vi "Upper Target Loop.vi"(11 "Camera Name":string="cam0") -> ()   [LabVIEW 2020]
uses:
  Camera Types.ctl
  Utilities/Camera Setup Cluster.ctl
  <vilib>/vision/Image Controls.llb/IMAQ Image.ctl
  Camera Set Up/Event Setup Types.ctl
  <vilib>/Utility/config.llb/Write Key (String).vi
  <vilib>/Utility/config.llb/Read Key (String).vi
  <vilib>/vision/NI_Vision_Development_Module.lvlib
  <vilib>/Utility/config.llb/NI_LVConfig.lvlib
panel:
  in  "Main":enum32{"Page 1", "Page 2"}(tab)
  in  "Configure":bool
  in  "Brightness":i32=50 min=0 max=100
  in  "Camera":enum32{"Mask", "Image With Target"}(tab)
  out "Mask":T1(plugin-control)
  out "Image":T1(plugin-control)
  in  "Save":bool
  out "Angle Array":dbl[](array[numeric]) format="%.1f"
  out "Distance  Array":dbl[](array[numeric]) format="%.1f"
  in  "White Balance":T2(ring)=enum."Fixed indoor"
  in  "FOV":dbl=120.0
  in  "Size Limit %":dbl=0.02 format="%#_13g"
  in  "Home":bool
  in  "Color Range":T3={"Hue"={21.620689392089844, 69.62068939208984}, "Sat"={66.41378784179688, 255.0}, "Val"={96.0, 255.0}} {"Hue" scale=0.0..255.0 scale format="%#_3g"}
  out "Fps":dbl format="%#.0f"
  in  "Camera Type":T4=enum."MS HD3000 640x480"
  in  "Dilate":bool
  in  "Robot Calibration":T5={"Camera Height on robot (in)"=26.7, "Camera Angle on the robot (deg)"=21.6, "Slope"=0.946, "Offset"=10.775} {"Offset" format="%#_13g"; "Slope" format="%#_13g"; "Camera Angle on the robot (deg)" format="%#_13g"; "Camera Height on robot (in)" format="%#_13g"}
  in  "Camera Exposure":i64=50 min=1 max=100
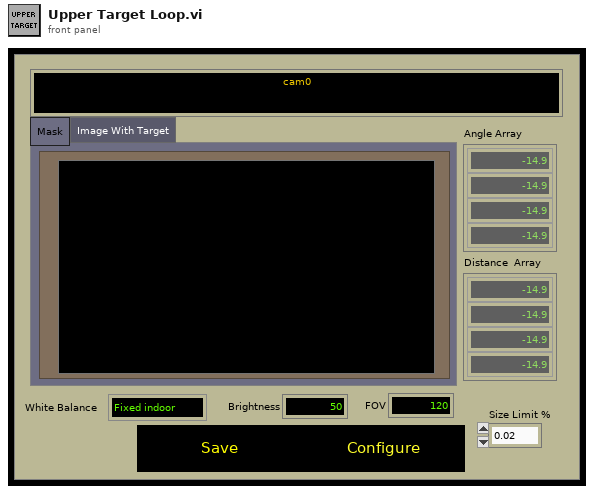
[diagram p1: front panel]
types:
  T1 = typedef "IMAQ Image.ctl" = refnum<image>
  T2 = enum16{"Auto", "Fixed indoor", "Fixed outdoor 1", "Fixed outdoor 2", "Fixed fluorescent 1", "Fixed fluorescent 2", "Hold current", "Custom"}
  T3 = cluster{"Hue":cluster{dbl, dbl}, "Sat":cluster{dbl, dbl}, "Val":cluster{dbl, dbl}}
  T4 = typedef "Camera Types.ctl" = enum16{"206", "1011", "1013", "MS HD3000 square", "MS HD3000 640x480", "MS HD3000 1280x720"}
  T5 = typedef "Camera Setup Cluster.ctl" = cluster{"Camera Height on robot (in)":dbl, "Camera Angle on the robot (deg)":dbl, "Slope":dbl, "Offset":dbl}
  T6 = typedef "Image Type" = u32
  T7 = typedef "Particle Parameters" = i32
  T8 = enum32{"AutoM", "Close", "Dilate", "Erode", "Gradient", "Gradient out", "Gradient in", "Hit miss", "Open", "PClose", "POpen", "Thick", "Thin"}
  T9 = typedef "Event Setup Types.ctl" = enum16{"Save Data", "Calibrate", "Set White Balance", "Set Brightness", "Set Exposure", "Update Brightness", "Update Exposure", "Update White Balance", "Exit"}
  T10 = typedef "Target Fields.ctl" = cluster{"diameter points":cluster{"first point":cluster{"x":dbl, "y":dbl}, "projected point":cluster{"x":dbl, "y":dbl}}, "normalized center":cluster{"x":dbl, "y":dbl}, "Overall Score":dbl, "Area Score":dbl, "Moment Score":dbl, "Aspect Score":dbl, "Distance (ft)":dbl, "Upper Goal":bool}
  T11 = typedef "NI_LVConfig.lvlib/Config Data RefNum.ctl" = refnum<k1>
  T12 = cluster{cluster{"Lower":dbl, "Upper":dbl}, cluster{"Lower":dbl, "Upper":dbl}, cluster{"Lower":dbl, "Upper":dbl}}
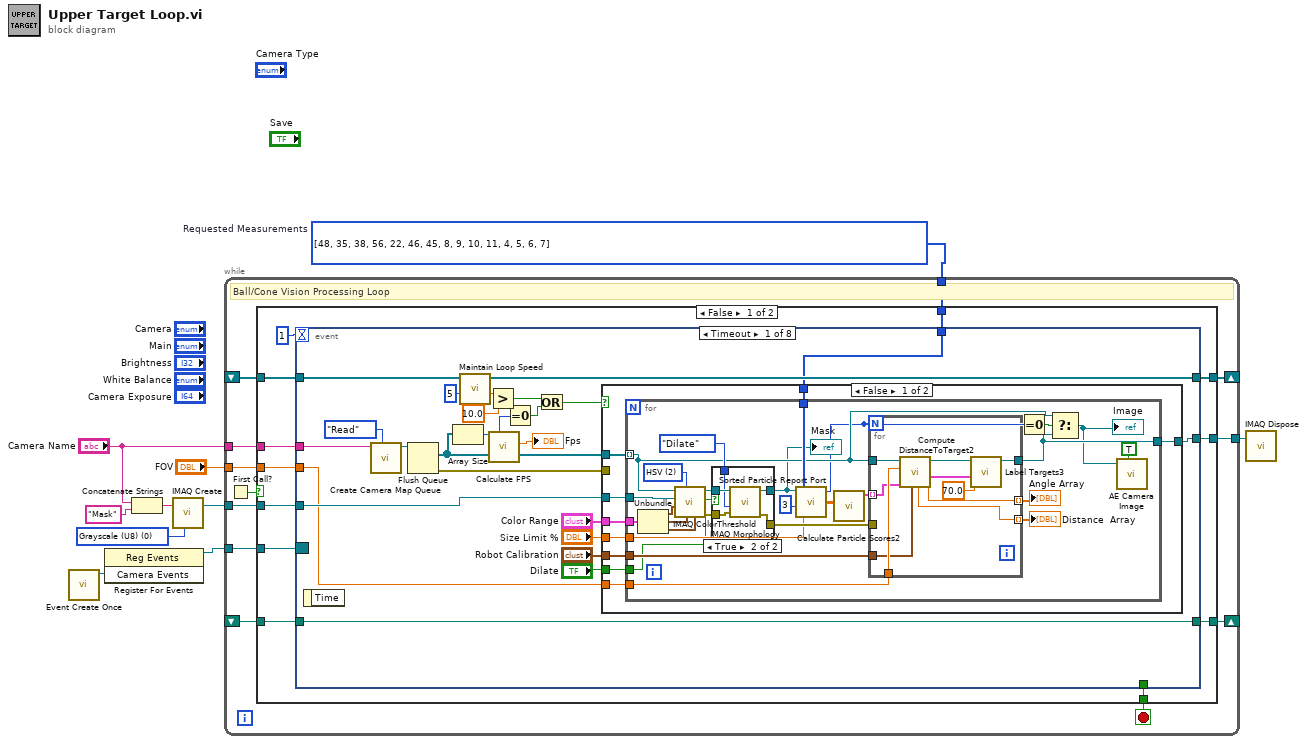
[diagram p0: block diagram]
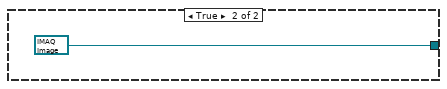
[diagram p3: hidden frame]
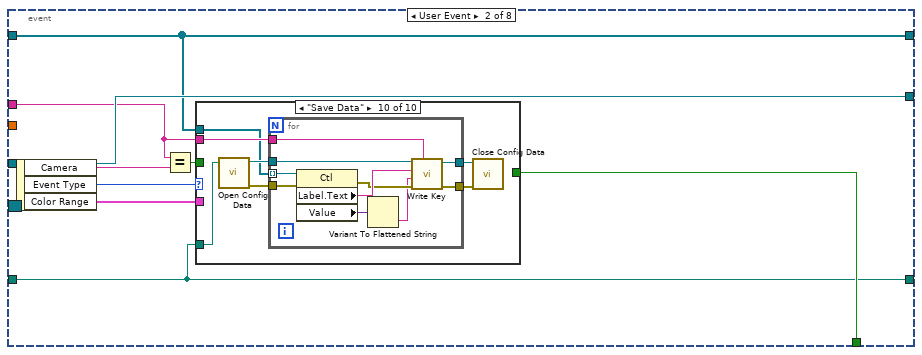
[diagram p4: hidden frame]
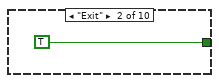
[diagram p6: hidden frame]
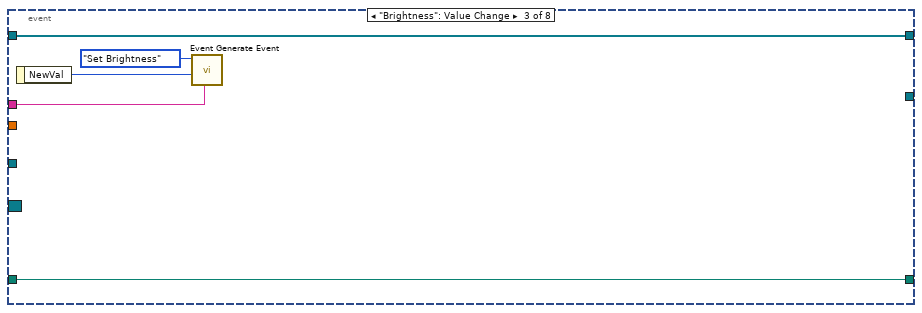
[diagram p14: hidden frame]
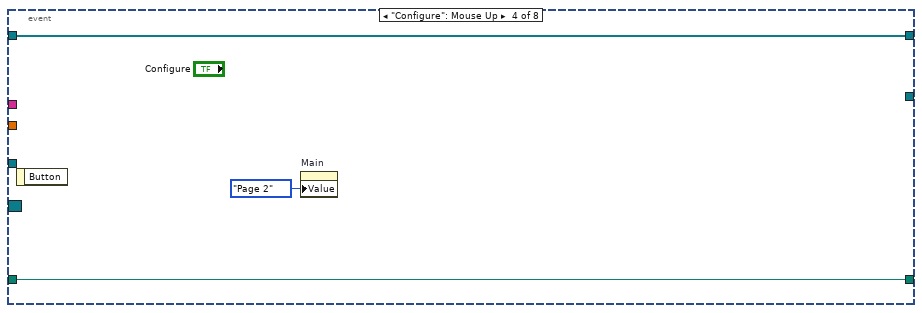
[diagram p15: hidden frame]
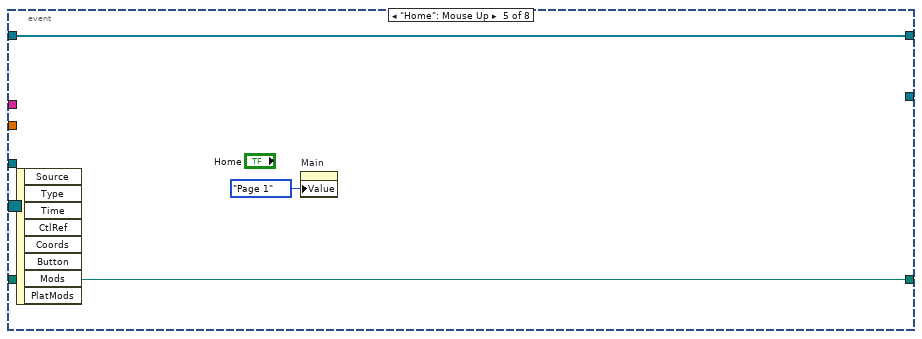
[diagram p16: hidden frame]
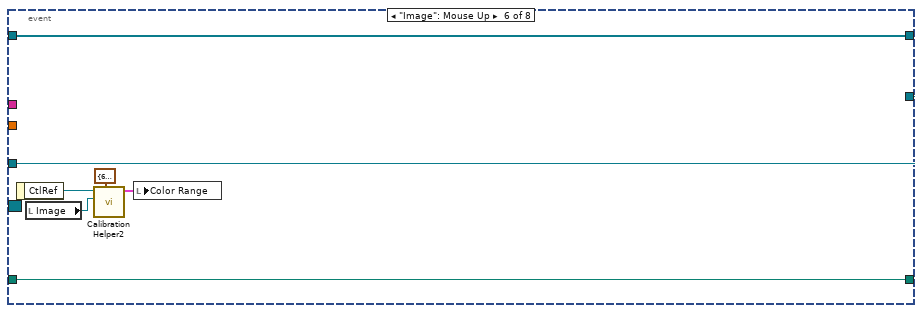
[diagram p17: hidden frame]
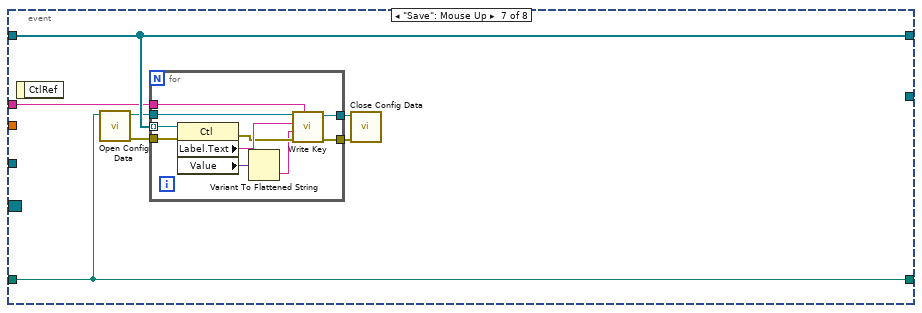
[diagram p18: hidden frame]
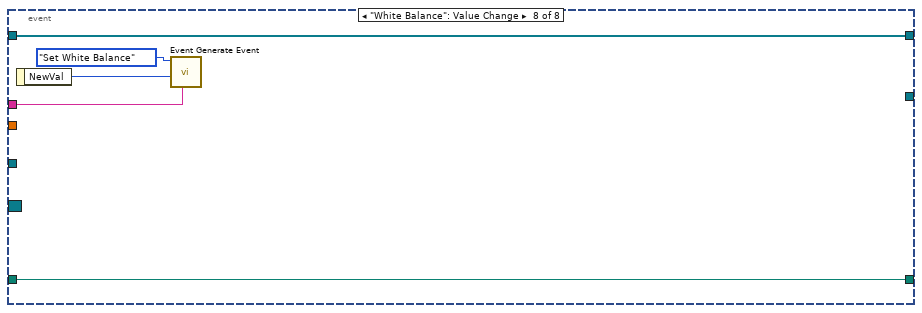
[diagram p19: hidden frame]
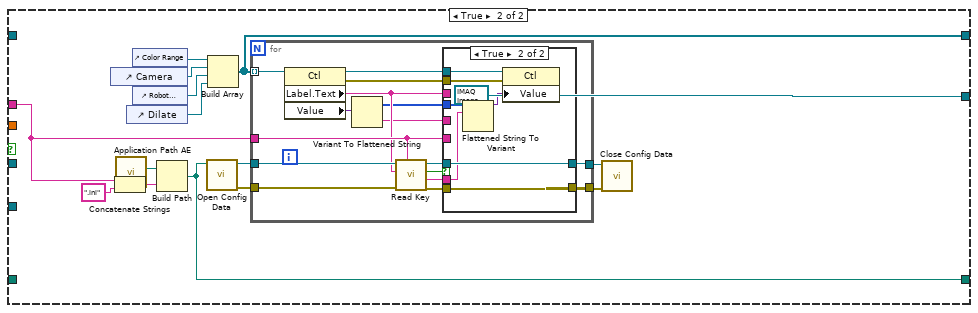
[diagram p20: hidden frame]
diagram:
  w6 = T6 0 items=["Grayscale (U8)", "Grayscale (I16)", "Grayscale (SGL)", "Complex (CSG)", "RGB (U32)", "HSL (U32)", "RGB (U64)", "Grayscale (U16)"] ("Image Type")
  w2 = T7[] [48, 35, 38, 56, 22, 46, 45, 8, 9, 10, 11, 4, 5, 6, 7] items=["Center of Mass X", "Center of Mass Y", "First Pixel X", "First Pixel Y", "Bounding Rect Left", "Bounding Rect Top", "Bounding Rect Right", "Bounding Rect Bottom", "Max Feret Diameter Start X", "Max Feret Diameter Start Y", "Max Feret Diameter End X", "Max Feret Diameter End Y", "Max Horiz. Segment Length Left", "Max Horiz. Segment Length Right", "Max Horiz. Segment Length Row", "-", "Bounding Rect Width", "Bounding Rect Height", "Bounding Rect Diagonal", "Perimeter", "Convex Hull Perimeter", "Holes' Perimeter", "Max Feret Diameter", "Equivalent Ellipse Major Axis", "Equivalent Ellipse Minor Axis", "Equivalent Ellipse Minor Axis (Feret)", "Equivalent Rect Long Side", "Equivalent Rect Short Side", "Equivalent Rect Diagonal", "Equivalent Rect Short Side (Feret)", "Average Horiz. Segment Length", "Average Vert. Segment Length", "Hydraulic Radius", "Waddel Disk Diameter", "-", "Area", "Holes' Area", "Particle & Holes' Area", "Convex Hull Area", "Image Area", "-", "Number of Holes", "Number of Horiz. Segments", "Number of Vert. Segments", "-", "Orientation", "Max Feret Diameter Orientation", "-", "% Area/Image Area", "% Area/(Particle & Holes' Area)", "Ratio of Equivalent Ellipse Axes", "Ratio of Equivalent Rect Sides", "-", "Elongation Factor", "Compactness Factor", "Heywood Circularity Factor", "Type Factor", "-", "Sum X", "Sum Y", "Sum XX", "Sum XY", "Sum YY", "Sum XXX", "Sum XXY", "Sum XYY", "Sum YYY", "-", "Moment of Inertia XX", "Moment of Inertia XY", "Moment of Inertia YY", "Moment of Inertia XXX", "Moment of Inertia XXY", "Moment of Inertia XYY", "Moment of Inertia YYY", "Norm. Moment of Inertia XX", "Norm. Moment of Inertia XY", "Norm. Moment of Inertia YY", "Norm. Moment of Inertia XXX", "Norm. Moment of Inertia XXY", "Norm. Moment of Inertia XYY", "Norm. Moment of Inertia YYY", "Hu Moment 1", "Hu Moment 2", "Hu Moment 3", "Hu Moment 4", "Hu Moment 5", "Hu Moment 6", "Hu Moment 7"]  # Requested Measurements
  n1 = call "Event Create Once.vi"() -> ("Camera Events"=w8:refnum<user-event>)  [unwired: 10 in, 1 out]
  n2 = register-events(w8) -> (reference out=w7:refnum<event-registration>)  [unwired: 2 in, 1 out]
  n3 = Concatenate Strings("Camera Name", "Mask" ("string")) -> (w5:string)
  n4 = call "IMAQ Create"("Image Name"=w5, "Image Type"=w6) -> ("New Image"=w10:T1)  [unwired: 2 in, 2 out]
  n5 = while {
    tunnel: w10 -> [w22]
    tunnel: w2 -> [w21]
    tunnel: [w20] -> w9
    tunnel: w7 -> [w19]
    tunnel: "FOV" -> [w17]
    tunnel: "Camera Name" -> [w16]
    shift-right: [w14] -> _
    shift-left: _ -> [w13]
    shift-right: [w12] -> _
    shift-left: _ -> [w11]
    stop <- w18 stop-if-true
    # "Ball/Cone Vision Processing Loop"
    n6 = First Call?() -> (First Call?: T/F=w15:bool)
    n7 = case shown="False" w15 {
      tunnel: w22 -> [w34 _]
      tunnel: w21 -> [w33 _]
      tunnel: [w32 T1 refnum ("New Image")] -> w20
      tunnel: w19 -> [w30 _]
      tunnel: [w29 _] -> w18
      tunnel: w17 -> [w28 _]
      tunnel: w16 -> [w27 w187]
      tunnel: [w25 w186] -> w14
      tunnel: w13 -> [w26 _]
      tunnel: [w23 w185] -> w12
      tunnel: w11 -> [w24 _]
      frame False {
        n8 = event shown="[0] Timeout" {
          selector: w30 -> [_ _ _ _ _ _ _ _]
          dyn-events: _ -> [_ _ _ _ _ _ _ _]
          timeout: 1 -> [_ _ _ _ _ _ _ _]
          tunnel: w34 -> [w51 w120 _ _ _ w154 _ _]
          tunnel: w33 -> [w49 _ _ _ _ _ _ _]
          tunnel: [w47 w120 _ _ _ w154 _ _] -> w32
          tunnel: [_ w118 _ _ _ _ _ _] -> w29
          tunnel: w28 -> [w50 _ _ _ _ _ _ _]
          tunnel: w27 -> [w56 w114 w141 _ _ _ w161 w176]
          tunnel: w26 -> [w55 w112 w140 w146 w149 w153 w162 w175]
          tunnel: [w55 w112 w140 w146 w149 w153 w162 w175] -> w25
          tunnel: w24 -> [w54 w113 w139 w145 w148 w152 w163 w174]
          tunnel: [w54 w113 w139 w145 w148 w152 w163 w174] -> w23
          event Timeout {
            n9 = event-data() -> ()  [unwired: 1 in, 1 out]
            n10 = call "Create Camera Map Queue.vi"("Action"=enum16{"Read", "Write"}."Read", "key"=w56) -> ("value"=w41:refnum<queue>)  [unwired: 8 in, 1 out]
            n11 = Flush Queue(queue=w41) -> (remaining elements=w36:T1[], error out=w40:errorcluster)  [unwired: 1 in, 1 out]
            n12 = Array Size(array=w36) -> (size(s)=w39:i32)
            n13 = call "Maintain Loop Speed.vi"("setpoint (msec)"=5) -> ("Loop Time"=w44:dbl)  [unwired: 10 in]
            n14 = Greater?(x=w44, y=10.0) -> (0:w45:bool)
            n15 = call "Calculate FPS.vi"("Frames Processed"=w39) -> ("Fps"=→"Fps":dbl)  [unwired: 10 in]
            n16 = Equal To 0?(x=w39) -> (x = 0?=w46:bool)
            n17 = Or(x=w45, y=w46) -> (x .or. y?=w35:bool)
            n18 = case shown="False" w35 {
              tunnel: w49 -> [w66 _]
              tunnel: w51 -> [w65 _]
              tunnel: [w60 T1 refnum ("Image out")] -> w47
              tunnel: "Color Range" -> [w64 _]
              tunnel: "Size Limit %" -> [w63 _]
              tunnel: "Robot Calibration" -> [w62 _]
              tunnel: w50 -> [w61 _]
              tunnel: "Dilate" -> [w59 _]
              tunnel: w36 -> [w58 _]
              tunnel: w40 -> [_ _]
              frame False {
                n19 = for {
                  tunnel: w66 -> [w93]
                  tunnel: w65 -> [w89]
                  tunnel: [w85] -> w60
                  tunnel: w58 -> [w78] mode=indexing
                  tunnel: w64 -> [w77]
                  tunnel: w63 -> [w76]
                  tunnel: w62 -> [w75]
                  tunnel: w61 -> [w74]
                  tunnel: w59 -> [w71]
                  w83 = u16 2 items=["RGB", "HSL", "HSV", "HSI"] ("Color Mode")
                  n20 = Unbundle(w77) -> ("Hue"=w90:cluster{dbl, dbl}, "Sat"=w92:cluster{dbl, dbl}, "Val"=w91:cluster{dbl, dbl})
                  n21 = call "IMAQ ColorThreshold"("Blue or Luma or Val or Inten Range"=w91, "Green or Sat Range"=w92, "Color Mode"=w83, "Red or Hue Range"=w90, "Image Dst"=w89, "Image Src"=w78) -> ("error out"=w80:errorcluster, "Image Dst Out"=w82:T1)  [unwired: 4 in]
                  n22 = case shown="True" w71 {
                    tunnel: w82 -> [w95 w100]
                    tunnel: [w95 w99] -> w70
                    tunnel: T8."Dilate" ("Operation") -> [_ w98]
                    tunnel: w80 -> [w94 w97]
                    tunnel: [w94 w96] -> w79
                    frame False {
                    }
                    frame True {
                      n23 = call "IMAQ Morphology"("error in (no error)"=w97, "Operation"=w98, "Image Src"=w100) -> ("error out"=w96:errorcluster, "Image Dst Out"=w99:T1)  [unwired: 7 in]
                    }
                  }
                  "Mask" <- w70
                  n24 = call "Sorted Particle Report Port.vi"("Min Area Size %"=w76, "Particle Count Limit"=3 ("Particle Count"), "Pixel Measurements"=w93, "Image in"=w70) -> ("Sorted Data"=w87:dbl[][], "Particles"=w73:i32)  [unwired: 1 out]
                  n25 = call "Calculate Particle Scores2.vi"("Sorted Data"=w87) -> ("Scores"=w86:T10[])  [unwired: 10 in]
                  n26 = for {
                    N: w73 -> [_]
                    tunnel: w86 -> [w105] mode=indexing
                    tunnel: [w104] -> w68 mode=indexing
                    tunnel: w74 -> [w106]
                    tunnel: w75 -> [w103]
                    tunnel: w79 -> [_]
                    tunnel: w78 -> [w109]
                    tunnel: [w110] -> w85
                    tunnel: [w101] -> w67 mode=indexing
                    n27 = call "Compute DistanceToTarget2.vi"("Robot Calibration Cluster"=w103, "results"=w105, "Field of view"=w106, "Image Src"=w109) -> ("results out"=w107:T10, "Offset Angle"=w104:dbl, "Image Dst Out"=w108:T1, "DIstance"=w101:dbl)  [unwired: 3 in, 1 out]
                    n28 = call "Label Targets3.vi"("Score Threshold"=70.0 ("Score Threshold %"), "results"=w107, "Image in"=w108) -> ("Image out"=w110:T1)  [unwired: 8 in]
                  }
                  "Angle Array" <- w68
                  "Distance  Array" <- w67
                  n29 = Equal To 0?(x=w73) -> (x = 0?=w84:bool)
                  n30 = Select(t=w78, s=w84, f=w85) -> (s? t:f=w69:T1)
                  "Image" <- w69
                  n31 = call "AE Camera Image.vi"("Update"=TRUE, "Upper Image in"=w69) -> ()  [unwired: 9 in, 1 out]
                }
              }
              frame True {
              }
            }
          }
          event User Event {
            n32 = event-data() -> ("Camera"=w115:string, "Event Type"=w119:T9, "Color Range"=w116:T3)  [unwired: 1 in]
            n33 = Equal?(x=w114, y=w115) -> (x = y?=w117:bool)
            n34 = case shown="\"Save Data\"" w119 {
              tunnel: [_ TRUE _ _ _ _ _ _ _ _] -> w118
              tunnel: w117 -> [_ _ _ _ _ _ _ _ _ _]
              tunnel: w116 -> [_ _ _ _ _ _ _ _ _ _]
              tunnel: w114 -> [_ _ _ _ _ _ _ _ _ w124]
              tunnel: w113 -> [_ _ _ _ _ _ _ _ _ w123]
              tunnel: w112 -> [_ _ _ _ _ _ _ _ _ w122]
              frame Default {
              }
              frame "Exit" {
              }
              frame "Update White Balance" {
              }
              frame "Update Exposure" {
              }
              frame "Update Brightness" {
              }
              frame "Set Exposure" {
              }
              frame "Set Brightness" {
              }
              frame "Set White Balance" {
              }
              frame "Calibrate" {
              }
              frame "Save Data" {
                n35 = call <vilib>:"Open Config Data.vi"("configuration file path"=w123) -> ("error out"=w125:errorcluster, "refnum"=w128:T11)  [unwired: 8 in, 1 out]
                n36 = for {
                  tunnel: w122 -> [w136] mode=indexing
                  tunnel: w128 -> [w138]
                  tunnel: w124 -> [w137]
                  tunnel: [w133] -> w127
                  tunnel: [w131] -> w126
                  tunnel: w125 -> [w130]
                  n37 = property class="Ctl"(reference=w136, error in=w130) -> (error out=w132:errorcluster, "Label.Text"=w135:string, "Value"=w134:variant)  [unwired: 1 out]
                  n38 = Variant To Flattened String(Variant=w134) -> (data string=w129:string)  [unwired: 1 out]
                  n39 = call-poly <vilib>:"Write Key.vi"("section"=w137, "error in (no error)"=w132, "value"=w129, "key"=w135, "refnum"=w138) -> ("error out"=w131:errorcluster, "refnum out"=w133:T11)  [unwired: 4 in, 1 out]
                }
                n40 = call <vilib>:"Close Config Data.vi"("error in (no error)"=w126, "refnum"=w127) -> ()  [unwired: 8 in, 2 out]
              }
            }
          }
          event "Brightness": Value Change {
            n41 = event-data() -> ("NewVal"=w142:i32)  [unwired: 1 in]
            n42 = call "Event Generate Event.vi"("Camera"=w141, "Setpoint"=w142, "Event Type"=Event_Setup_Types."Set Brightness") -> ()  [unwired: 9 in]
          }
          event "Configure": Mouse Up {
            n43 = event-data() -> ()  [unwired: 1 in, 1 out]
            n44 = property on="Main" class="TabCtl (strict)"("Value"=enum32{"Page 1", "Page 2"}."Page 2" ("Main")) -> ()  [unwired: 2 in, 2 out]
          }
          event "Home": Mouse Up {
            n45 = event-data() -> ()  [unwired: 1 in, 8 out]
            n46 = property on="Main" class="TabCtl (strict)"("Value"=enum32{"Page 1", "Page 2"}."Page 1" ("Main")) -> ()  [unwired: 2 in, 2 out]
          }
          event "Image": Mouse Up {
            n47 = event-data() -> ("CtlRef"=w151:refnum<vi>)  [unwired: 1 in]
            n48 = local read "Image"() -> (w150:T1)
            n49 = call "Calibration Helper2.vi"("Std Devs"=cluster{"H":dbl, "S":dbl, "V":dbl} {"H"=6.0, "S"=6.0, "V"=6.0} ("Std Devs Ball"), "Image"=w150, "Image Ctl Refnum"=w151) -> ("output color"=w155:T12)  [unwired: 7 in, 1 out]
            n50 = local write "Color Range"(w155) -> ()
          }
          event "Save": Mouse Up {
            n51 = event-data() -> ()  [unwired: 1 in, 1 out]
            n52 = call <vilib>:"Open Config Data.vi"("configuration file path"=w163) -> ("error out"=w157:errorcluster, "refnum"=w160:T11)  [unwired: 8 in, 1 out]
            n53 = for {
              tunnel: w162 -> [w171] mode=indexing
              tunnel: w160 -> [w173]
              tunnel: w161 -> [w172]
              tunnel: [w168] -> w159
              tunnel: [w166] -> w158
              tunnel: w157 -> [w165]
              n54 = property class="Ctl"(reference=w171, error in=w165) -> (error out=w167:errorcluster, "Label.Text"=w170:string, "Value"=w169:variant)  [unwired: 1 out]
              n55 = Variant To Flattened String(Variant=w169) -> (data string=w164:string)  [unwired: 1 out]
              n56 = call-poly <vilib>:"Write Key.vi"("section"=w172, "error in (no error)"=w167, "value"=w164, "key"=w170, "refnum"=w173) -> ("error out"=w166:errorcluster, "refnum out"=w168:T11)  [unwired: 4 in, 1 out]
            }
            n57 = call <vilib>:"Close Config Data.vi"("error in (no error)"=w158, "refnum"=w159) -> ()  [unwired: 8 in, 2 out]
          }
          event "White Balance": Value Change {
            n58 = event-data() -> ("NewVal"=w177:T2)  [unwired: 1 in]
            n59 = call "Event Generate Event.vi"("Camera"=w176, "Setpoint"=w177, "Event Type"=Event_Setup_Types."Set White Balance") -> ()  [unwired: 9 in]
          }
        }
      }
      frame True {
        n60 = control-ref of="Camera"() -> (w182:refnum<vi>)
        n61 = Concatenate Strings(w187, ".ini" ("name or relative path")) -> (w192:string)
        n62 = call "Application Path AE.vi"() -> ("Application Path out"=w179:path)  [unwired: 11 in]
        n63 = control-ref of="Dilate"() -> (w180:refnum<vi>)
        n64 = control-ref of="Color Range"() -> (w183:refnum<vi>)
        n65 = control-ref of="Robot Calibration"() -> (w181:refnum<vi>)
        n66 = Build Path(base path=w179, name or relative path=w192) -> (appended path=w185:path)
        n67 = call <vilib>:"Open Config Data.vi"("configuration file path"=w185) -> ("error out"=w184:errorcluster, "refnum"=w191:T11)  [unwired: 8 in, 1 out]
        n68 = Build Array(w183, w182, w181, w180) -> (w186:refnum<vi>[])
        n69 = for {
          tunnel: w191 -> [w209]
          tunnel: w187 -> [w202]
          tunnel: w186 -> [w208] mode=indexing
          tunnel: [w200] -> w190
          tunnel: [w198] -> w189
          tunnel: w184 -> [w194]
          n70 = property class="Ctl"(reference=w208) -> (reference out=w205:refnum<vi>, error out=w204:errorcluster, "Label.Text"=w201:string, "Value"=w197:variant)  [unwired: 1 in]
          n71 = Variant To Flattened String(Variant=w197) -> (data string=w196:string, 1:w195:i16[])
          n72 = call-poly <vilib>:"Read Key.vi"("section"=w202, "error in (no error)"=w194, "key"=w201, "refnum"=w209) -> ("error out"=w199:errorcluster, "value"=w206:string, "found?"=w207:bool, "refnum out"=w203:T11)  [unwired: 4 in]
          n73 = case shown="True" w207 {
            tunnel: w206 -> [_ w218]
            tunnel: w205 -> [_ w223]
            tunnel: w204 -> [_ w222]
            tunnel: w203 -> [w216 w221]
            tunnel: w202 -> [w215 _]
            tunnel: w201 -> [w214 _]
            tunnel: [w213 w221] -> w200
            tunnel: w199 -> [w212 w220]
            tunnel: [w211 w220] -> w198
            tunnel: w196 -> [w210 _]
            tunnel: w195 -> [_ w219]
            frame False {
              n74 = call-poly <vilib>:"Write Key.vi"("section"=w215, "error in (no error)"=w212, "value"=w210, "key"=w214, "refnum"=w216) -> ("error out"=w211:errorcluster, "refnum out"=w213:T11)  [unwired: 4 in, 1 out]
            }
            frame True {
              n75 = Flattened String To Variant(6:w218, 7:w219) -> (3:w217:variant)  [unwired: 1 in, 1 out]
              n76 = property class="Ctl"(reference=w223, error in=w222, "Value"=w217) -> ()  [unwired: 2 out]
            }
          }
        }
        n77 = call <vilib>:"Close Config Data.vi"("error in (no error)"=w189, "refnum"=w190) -> ()  [unwired: 8 in, 2 out]
      }
    }
  }
  n78 = call "IMAQ Dispose"("Image"=w9) -> ()  [unwired: 5 in, 1 out]
